vi "MGI Button Dialog.vi"(0 "Hide calling VI? (FALSE)":bool, 4 "Allow user to close window? (TRUE)":bool=TRUE, 5 "Justify Message (Left)":enum16{"Left", "Center", "Right"}(ring), 6 "Keyboard Shortcuts (Left is <Enter>)":T2={"Left Button Key Shortcut"={"Control"=FALSE, "Shift"=FALSE, "Key"="<Enter>"}, "Center Button Key Shortcut"={"Control"=FALSE, "Shift"=FALSE, "Key"=""}, "Right Button Key Shortcut"={"Control"=FALSE, "Shift"=FALSE, "Key"="<Escape>"}}, 7 "Window Title (\"\")":string, 8 "Right Button Text (\"Cancel\")":string="Cancel", 9 "Center Button Text (\"\":hidden)":string, 10 "Left Button Text (\"OK\")":string="OK", 11 "Message":string) -> (2 "Left Button?":bool, 3 "Which Button?":T1(ring)=enum."Center Button")   [LabVIEW 2020]
doc: "Enhanced version of the built in three button dialog for original help, click link below).\n\nAdded an output boolean useful for drop-in replacement of one- or two-button dialogs, which as in the original you'll get by wiring empty strings for button text. Added an option to make this a non-modal dialog but hide the calling VI, which is useful when you want to block one window but not all windows. This VI is reentrant to support that situation.\n\nAuthored by David A. Moore\nsupport@mooregoodideas.com\nwww.mooregoodideas.com\n\nCopyright (c) 2010, Moore Good Ideas, Inc.\n\nAll rights reserved.\n\nRedistribution and use in source and binary forms, with or without modification, are permitted provided that the following conditions are met:\n\n * Redistributions of source code must retain the above copyright notice, this list of conditions and the following disclaimer.\n * Redistributions in binary form must reproduce the above copyright notice, this list of conditions and the following disclaimer in the documentation and/or other materials provided with the distribution.\n * Neither the name of Moore Good Ideas, Inc. nor the names of its contributors may be used to endorse or promote products derived from this software without specific prior written permission.\n\nTHIS SOFTWARE IS PROVIDED BY THE COPYRIGHT HOLDERS AND CONTRIBUTORS \"AS IS\" AND ANY EXPRESS OR IMPLIED WARRANTIES, INCLUDING, BUT NOT LIMITED TO, THE IMPLIED WARRANTIES OF MERCHANTABILITY AND FITNESS FOR A PARTICULAR PURPOSE ARE DISCLAIMED. IN NO EVENT SHALL THE COPYRIGHT OWNER OR CONTRIBUTORS BE LIABLE FOR ANY DIRECT, INDIRECT, INCIDENTAL, SPECIAL, EXEMPLARY, OR CONSEQUENTIAL DAMAGES (INCLUDING, BUT NOT LIMITED TO, PROCUREMENT OF SUBSTITUTE GOODS OR SERVICES; LOSS OF USE, DATA, OR PROFITS; OR BUSINESS INTERRUPTION) HOWEVER CAUSED AND ON ANY THEORY OF LIABILITY, WHETHER IN CONTRACT, STRICT LIABILITY, OR TORT (INCLUDING NEGLIGENCE OR OTHERWISE) ARISING IN ANY WAY OUT OF THE USE OF THIS SOFTWARE, EVEN IF ADVISED OF THE POSSIBILITY OF SUCH DAMAGE."
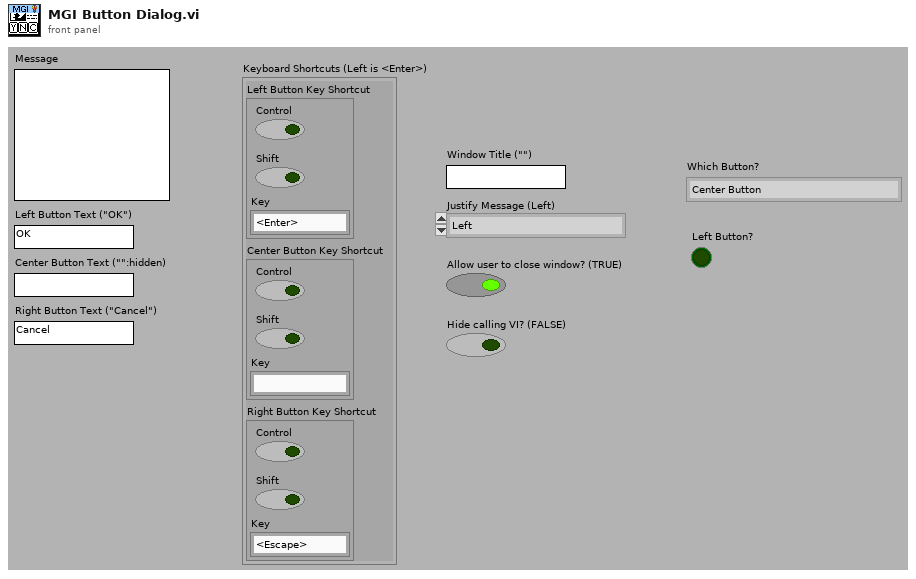
[diagram p1: front panel]
types:
  T1 = enum16{"Left Button", "Center Button", "Right Button", "Window Close"}
  T2 = cluster{"Left Button Key Shortcut":cluster{"Control":bool, "Shift":bool, "Key":string}, "Center Button Key Shortcut":cluster{"Control":bool, "Shift":bool, "Key":string}, "Right Button Key Shortcut":cluster{"Control":bool, "Shift":bool, "Key":string}}
  T3 = enum32{"Invalid", "Default", "Floating", "Floating/Auto-Hide", "Modal"}
  T4 = enum32{"Invalid", "Standard", "Closed", "Hidden", "Minimized", "Maximized"}
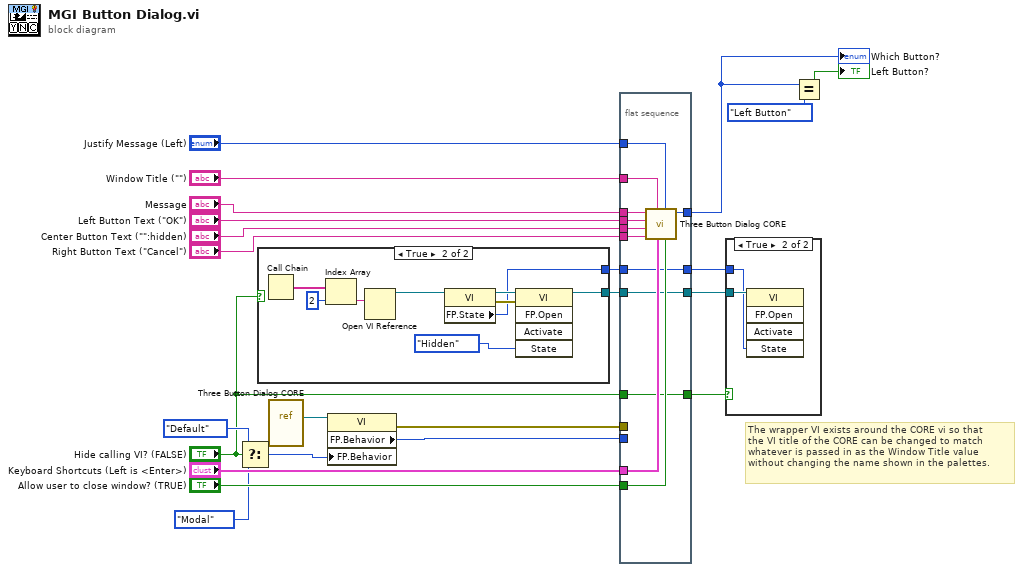
[diagram p0: block diagram]
diagram:
  # "The wrapper VI exists around the CORE vi so that\nthe VI title of the CORE can be changed to match\nwhatever is passed in as the Window Title value\nwithout changing the name shown in the palettes."
  n1 = Select(t=T3."Default" ("Front Panel Window:Behavior"), s="Hide calling VI? (FALSE)", f=T3."Modal" ("Front Panel Window:Behavior")) -> (s? t:f=w9:T3)
  n2 = case shown="True" "Hide calling VI? (FALSE)" {
    tunnel: [_ w29] -> w6
    tunnel: [_ w28] -> w4
    frame False {
    }
    frame True {
      n3 = Call Chain() -> (call chain=w27:string[])
      n4 = Index Array(array=w27, index=2) -> (element=w26:string)
      n5 = Open VI Reference(vi path=w26) -> (vi reference=w24:refnum<vi>)  [unwired: 5 in, 1 out]
      n6 = property class="VI"(reference=w24) -> (reference out=w31:refnum<vi>, error out=w32:errorcluster, "FP.State"=w29:T4)  [unwired: 1 in]
      n7 = invoke class="VI" method="FP.Open"(reference=w31, error in=w32, "State"=T4."Hidden") -> (reference out=w28:refnum<vi>)  [unwired: 2 in, 4 out]
    }
  }
  n8 = vi-ref <vilib>:"Three Button Dialog CORE.vi"() -> (w12:refnum<vi>)
  n9 = property class="VI"(reference=w12, "FP.Behavior"=w9) -> (error out=w8:errorcluster, "FP.Behavior"=w7:T3)  [unwired: 1 in, 1 out]
  n10 = flat-sequence {
    tunnel: "Window Title (\"\")" -> [w44]
    tunnel: "Justify Message (Left)" -> [w43]
    tunnel: [w42] -> w21
    tunnel: "Allow user to close window? (TRUE)" -> [w41]
    tunnel: "Keyboard Shortcuts (Left is <Enter>)" -> [w40]
    tunnel: "Right Button Text (\"Cancel\")" -> [w39]
    tunnel: "Center Button Text (\"\":hidden)" -> [w38]
    tunnel: "Left Button Text (\"OK\")" -> [w37]
    tunnel: "Message" -> [w36]
    tunnel: w8 -> [_]
    tunnel: w7 -> [_]
    tunnel: w6 -> [w34]
    tunnel: "Hide calling VI? (FALSE)" -> [w33]
    tunnel: w4 -> [w35]
    tunnel: [w35] -> w3
    tunnel: [w34] -> w2
    tunnel: [w33] -> w1
    frame #0 {
      n11 = call <vilib>:"Three Button Dialog CORE.vi"("Allow user to close window? (TRUE)"=w41, "Justify Message (Left)"=w43, "Keyboard Shortcuts (Left is <Enter>)"=w40, "Window Title (\"\")"=w44, "Right Button Text (\"Cancel\")"=w39, "Center Button Text (\"No\")"=w38, "Left Button Text (\"Yes\")"=w37, "message"=w36) -> ("Which Button?"=w42:T1)  [unwired: 3 in]
    }
  }
  n12 = case shown="True" w1 {
    tunnel: w3 -> [_ w46]
    tunnel: w2 -> [_ w45]
    frame False {
    }
    frame True {
      n13 = invoke class="VI" method="FP.Open"(reference=w46, "State"=w45) -> ()  [unwired: 3 in, 5 out]
    }
  }
  n14 = Equal?(x=w21, y=T1."Left Button") -> (x = y?=→"Left Button?":bool)
  "Which Button?" <- w21
